vi "testOption.vi"(8 "Error In":errorcluster, 10 "option":T1=1 items=["NoButtons"=1, "DontUseNativeDialog"=2, "ScalableFonts"=4, "NonScalableFonts"=8, "MonospacedFonts"=16, "ProportionalFonts"=32], 11 "QFontDialog In":refnum<class "QFontDialog.lvclass">) -> (0 "Error Out":errorcluster, 2 "Value":bool, 3 "QFontDialog Out":refnum<class "QFontDialog.lvclass">)   [LabVIEW 2014, in "QFontDialog.lvclass"]
doc: "LabVIEW-specific documentation is not yet available. See <b>https://doc.qt.io/qt-5/qfontdialog.html#testOption</b>"
uses:
  QFontDialog.lvclass
  FontDialogOption.ctl
  LQ Core/LQIdentity/LQIdentity.lvclass/LQIdentity.ctl
  LQ Core/LQ Core.lvlib
  LQ Core/LQIdentity/LQIdentity.lvclass
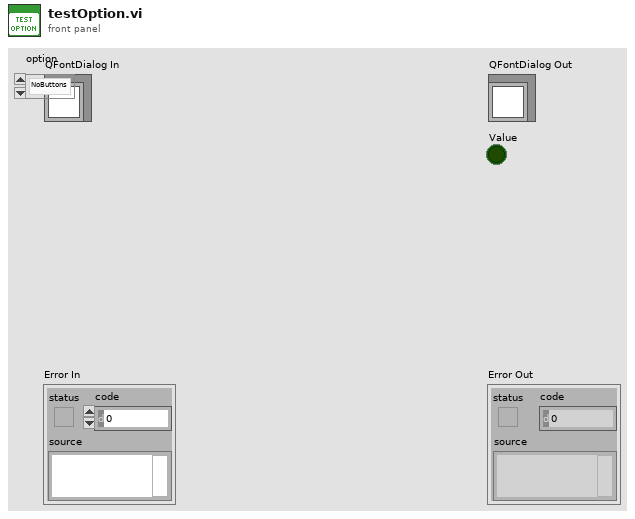
[diagram p1: front panel]
types:
  T1 = typedef "QFontDialog.lvclass/FontDialogOption.ctl" = i32
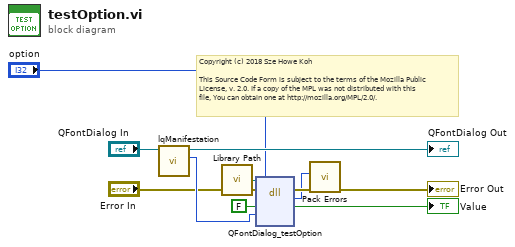
[diagram p0: block diagram]
diagram:
  # "Copyright (c) 2018 Sze Howe Koh\n\nThis Source Code Form is subject to the terms of the Mozilla Public\nLicense, v. 2.0. If a copy of the MPL was not distributed with this\nfile, You can obtain one at http://mozilla.org/MPL/2.0/."
  n1 = call "lqManifestation.vi"("LQIdentity in"="QFontDialog In") -> ("Manifestation"=w6:u64, "LQIdentity out"=→"QFontDialog Out":refnum<class "QFontDialog.lvclass">)  [unwired: 9 in]
  n2 = call "Library Path.vi"() -> ("Library Path"=w7:path)
  n3 = dll-call lib="?" fn="QFontDialog_testOption"(path in=w7, error in="Error In", "_retVal"=FALSE, "_instance"=w6, "option"="option") -> (error out=w4:errorcluster, w2:i32, "_retVal"=→"Value":bool)  [unwired: 3 in, 1 out]
  n4 = call "Pack Errors.vi"("Error In"=w4, "Error Code"=w2) -> ("Error Out"=→"Error Out":errorcluster)  [unwired: 9 in]
